vi "ImageComplexCsgToArray.vi"(8 "error in":errorcluster, 10 "Optional Rectangle":T1, 11 "Image Reference In":T2) -> (0 "error out":errorcluster, 2 "Pixel":csg[][](array[numeric]), 3 "Image Reference Out":T2)   [LabVIEW 2020, in "OpenLvVision_Image.lvlib" / "DataAccess.lvlib"]
doc: "Copies the pixel into an 2D array without an border."
uses:
  DataAccess.lvlib
  Management/TypeDef/Image.ctl
  TypeDef/RectangleI32.ctl
  Management/Management.lvlib
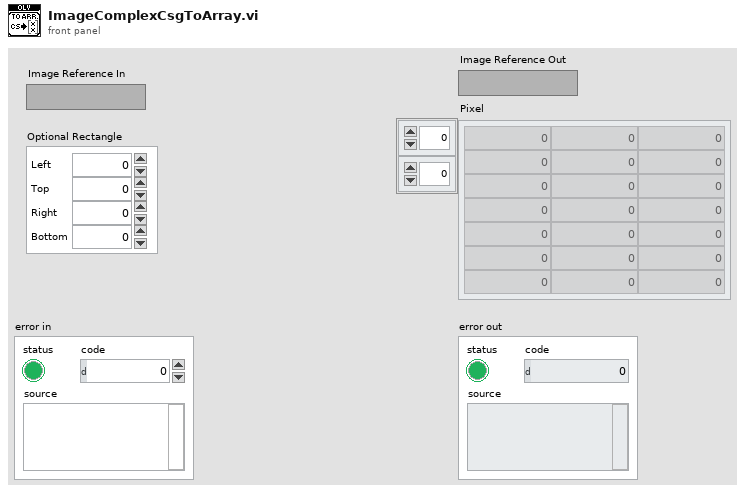
[diagram p1: front panel]
types:
  T1 = typedef "OpenLvVision_Image.lvlib/DataAccess.lvlib/RectangleI32.ctl" = cluster{"Left":i32, "Top":i32, "Right":i32, "Bottom":i32}
  T2 = typedef "OpenLvVision_Image.lvlib/Management.lvlib/Image.ctl" = refnum<image>
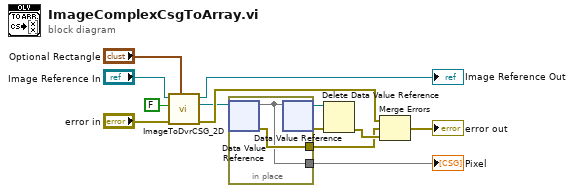
[diagram p0: block diagram]
diagram:
  n1 = call "ImageToDvrCSG_2D.vi"("Optional Rectangle"="Optional Rectangle", "error in"="error in", "Include Border"=FALSE, "Image Reference In"="Image Reference In") -> ("error out"=w11:errorcluster, "EDVR 2D CSG"=w10:refnum<data-value>, "Image Reference Out"=→"Image Reference Out":T2)  [unwired: 4 in, 1 out]
  n2 = in-place {
    in-place-border: [w15] -> w8
    in-place-border: [w14] -> w3
    n3 = in-place-dvr #1(w10) -> (w14:csg[][], w15:errorcluster)
    n4 = in-place-dvr #1(w14) -> (w12:refnum<data-value>, w13:errorcluster)
  }
  "Pixel" <- w3
  n5 = Delete Data Value Reference(data value reference=w12, error in=w13) -> (error out=w9:errorcluster)  [unwired: 1 out]
  n6 = Merge Errors(w11, w8, w9) -> (→"error out":errorcluster)
